vi "parameter e2n.vi"(1 "parameter":T1) -> (0 "number":u8 format="%x")   [LabVIEW 2024, in "atsj peakcan basic.lvlib"]
uses:
  atsj peakcan basic.lvlib
  parameter.ctl
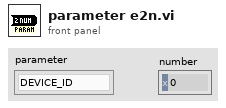
[diagram p1: front panel]
types:
  T1 = typedef "atsj peakcan basic.lvlib/parameter.ctl" = enum8{"DEVICE_ID", "5VOLTS_POWER", "RECEIVE_EVENT", "MESSAGE_FILTER", "API_VERSION", "CHANNEL_VERSION", "BUSOFF_AUTORESET", "LISTEN_ONLY", "LOG_LOCATION", "LOG_STATUS", "LOG_CONFIGURE", "LOG_TEXT", "CHANNEL_CONDITION", "HARDWARE_NAME", "RECEIVE_STATUS", "CONTROLLER_NUMBER", "TRACE_LOCATION", "TRACE_STATUS", "TRACE_SIZE", "TRACE_CONFIGURE", "CHANNEL_IDENTIFYING", "CHANNEL_FEATURES", "BITRATE_ADAPTING", "BITRATE_INFO", "BITRATE_INFO_FD", "BUSSPEED_NOMINAL", "BUSSPEED_DATA", "IP_ADDRESS", "LAN_SERVICE_STATUS", "ALLOW_STATUS_FRAMES", "ALLOW_RTR_FRAMES", "ALLOW_ERROR_FRAMES", "INTERFRAME_DELAY", "ACCEPTANCE_FILTER_11BIT", "ACCEPTANCE_FILTER_29BIT", "IO_DIGITAL_CONFIGURATION", "IO_DIGITAL_VALUE", "IO_DIGITAL_SET", "IO_DIGITAL_CLEAR", "IO_ANALOG_VALUE", "FIRMWARE_VERSION", "ATTACHED_CHANNELS_COUNT", "ATTACHED_CHANNELS", "ALLOW_ECHO_FRAMES", "DEVICE_PART_NUMBER", "HARD_RESET_STATUS", "LAN_CHANNEL_DIRECTION", "DEVICE_GUID"}
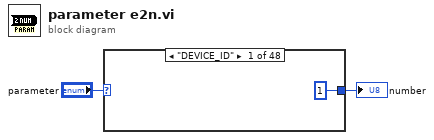
[diagram p0: block diagram]
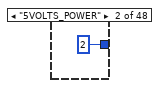
[diagram p2: hidden frame]
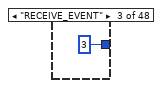
[diagram p3: hidden frame]
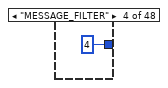
[diagram p4: hidden frame]
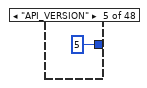
[diagram p5: hidden frame]
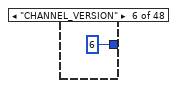
[diagram p6: hidden frame]
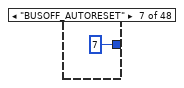
[diagram p7: hidden frame]
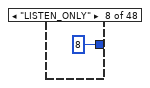
[diagram p8: hidden frame]
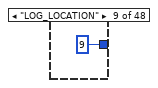
[diagram p9: hidden frame]
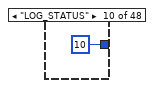
[diagram p10: hidden frame]
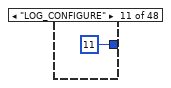
[diagram p11: hidden frame]
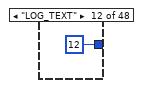
[diagram p12: hidden frame]
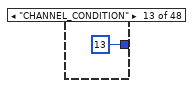
[diagram p13: hidden frame]
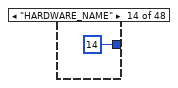
[diagram p14: hidden frame]
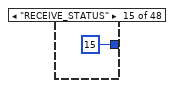
[diagram p15: hidden frame]
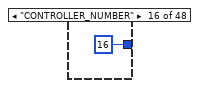
[diagram p16: hidden frame]
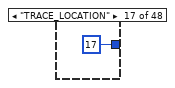
[diagram p17: hidden frame]
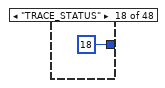
[diagram p18: hidden frame]
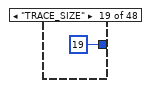
[diagram p19: hidden frame]
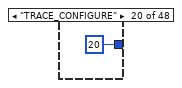
[diagram p20: hidden frame]
diagram:
  n1 = case shown="\"DEVICE_ID\"" "parameter" {
    tunnel: [u8 1 u8 2 u8 3 u8 4 u8 5 u8 6 u8 7 u8 8 u8 9 u8 10 u8 11 u8 12 u8 13 u8 14 u8 15 u8 16 u8 17 u8 18 u8 19 u8 20 u8 21 u8 22 u8 23 u8 24 u8 25 u8 26 u8 27 u8 28 u8 29 u8 30 u8 31 u8 32 u8 33 u8 34 u8 35 u8 36 u8 37 u8 38 u8 39 u8 40 u8 41 u8 42 u8 43 u8 44 u8 45 u8 46 u8 47 u8 48] -> w1
    frame "DEVICE_ID" {
    }
    frame "5VOLTS_POWER" {
    }
    frame "RECEIVE_EVENT" {
    }
    frame "MESSAGE_FILTER" {
    }
    frame "API_VERSION" {
    }
    frame "CHANNEL_VERSION" {
    }
    frame "BUSOFF_AUTORESET" {
    }
    frame "LISTEN_ONLY" {
    }
    frame "LOG_LOCATION" {
    }
    frame "LOG_STATUS" {
    }
    frame "LOG_CONFIGURE" {
    }
    frame "LOG_TEXT" {
    }
    frame "CHANNEL_CONDITION" {
    }
    frame "HARDWARE_NAME" {
    }
    frame "RECEIVE_STATUS" {
    }
    frame "CONTROLLER_NUMBER" {
    }
    frame "TRACE_LOCATION" {
    }
    frame "TRACE_STATUS" {
    }
    frame "TRACE_SIZE" {
    }
    frame "TRACE_CONFIGURE" {
    }
    frame "CHANNEL_IDENTIFYING" {
    }
    frame "CHANNEL_FEATURES" {
    }
    frame "BITRATE_ADAPTING" {
    }
    frame "BITRATE_INFO" {
    }
    frame "BITRATE_INFO_FD" {
    }
    frame "BUSSPEED_NOMINAL" {
    }
    frame "BUSSPEED_DATA" {
    }
    frame "IP_ADDRESS" {
    }
    frame "LAN_SERVICE_STATUS" {
    }
    frame "ALLOW_STATUS_FRAMES" {
    }
    frame "ALLOW_RTR_FRAMES" {
    }
    frame "ALLOW_ERROR_FRAMES" {
    }
    frame "INTERFRAME_DELAY" {
    }
    frame "ACCEPTANCE_FILTER_11BIT" {
    }
    frame "ACCEPTANCE_FILTER_29BIT" {
    }
    frame "IO_DIGITAL_CONFIGURATION" {
    }
    frame "IO_DIGITAL_VALUE" {
    }
    frame "IO_DIGITAL_SET" {
    }
    frame "IO_DIGITAL_CLEAR" {
    }
    frame "IO_ANALOG_VALUE" {
    }
    frame "FIRMWARE_VERSION" {
    }
    frame "ATTACHED_CHANNELS_COUNT" {
    }
    frame "ATTACHED_CHANNELS" {
    }
    frame "ALLOW_ECHO_FRAMES" {
    }
    frame "DEVICE_PART_NUMBER" {
    }
    frame "HARD_RESET_STATUS" {
    }
    frame "LAN_CHANNEL_DIRECTION" {
    }
    frame "DEVICE_GUID" {
    }
  }
  "number" <- w1
